vi "Timer_ISR.vi"(11 "TIMX_Interrupt":T1) -> ()   [LabVIEW 2011]
uses:
  D:/National Instruments/LabVIEW 2011/Targets/Keil/Embedded/RealView/Generic/My_ARM_Starter_Board_F4/STM32_DriverVI_Interface/Timer/Timer_ISR_F4.ctl
  <vilib>/eio/EIO_TerminalDirection.ctl
  <vilib>/STM32_DriverVI_Interface_F4/Timer/TIM5_Flag_F4.ctl
  <vilib>/STM32_DriverVI_Interface_F4/Timer/TIM5_Capture_Channel_F4.ctl
  <vilib>/STM32_DriverVI_Interface_F4/Timer/Edge Mode_F4.ctl
  <vilib>/STM32_DriverVI_Interface_F4/Timer/TIM5_Get_Channel_F4.ctl
  <vilib>/STM32_DriverVI_Interface_F4/GPIO_EIO/GPO_EIO_Inner_F4.vi
  <vilib>/STM32_DriverVI_Interface_F4/Timer/Clear_TIM5_Flag_F4.vi
  <vilib>/STM32_DriverVI_Interface_F4/Timer/TIM5 Channel Edge Set_F4.vi
  <vilib>/STM32_DriverVI_Interface_F4/Timer/TIM5_Set_Counter_F4.vi
  <vilib>/STM32_DriverVI_Interface_F4/Timer/TIM5 Get Channel_Value_F4.vi
  <vilib>/eio/EIONode/EIONode.xnode
panel:
  # "这是一个标准的中断模板 VI，用户可以直接使用,\n在相应的Case语句里面实现相应的中断服务程序即可！\n\n双击打开这个VI之后，另存为副本，名称不变，将其保存\n并添加到项目浏览器中，然后在程序生成规范中进行属性\n设置！"
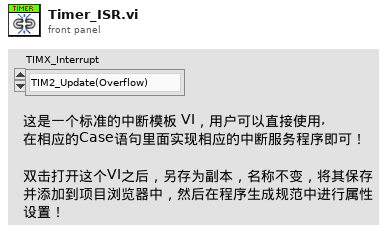
[diagram p1: front panel]
types:
  T1 = typedef "Timer_ISR_F4.ctl" = enum8{"TIM2_Update(Overflow)", "TIM2_Channel_1", "TIM2_Channel_2", "TIM2_Channel_3", "TIM2_Channel_4", "TIM3_Update(Overflow)", "TIM3_Channel_1", "TIM3_Channel_2", "TIM3_Channel_3", "TIM3_Channel_4", "TIM4_Update(Overflow)", "TIM4_Channel_1", "TIM4_Channel_2", "TIM4_Channel_3", "TIM4_Channel_4", "TIM5_Update(Overflow)", "TIM5_Channel_1", "TIM5_Channel_2", "TIM5_Channel_3", "TIM5_Channel_4", "TIM6_Update(Overflow)", "TIM7_Update(Overflow)", "----------------------------", "WWDG_ISR", "RTC_Alarm_ClockA_ISR", "RTC_Alarm_ClockB_ISR", "RTC_WKUP_ISR", "TIM1_Update(Overflow)", "TIM1_Channel_1", "TIM1_Channel_2", "TIM1_Channel_3", "TIM1_Channel_4", "TIM8_Update(Overflow)", "TIM8_Channel_1", "TIM8_Channel_2", "TIM8_Channel_3", "TIM8_Channel_4", "TIM9_Update(Overflow)", "TIM9_Channel_1", "TIM9_Channel_2", "TIM10_Update(Overflow)", "TIM10_Channel_1", "TIM11_Update(Overflow)", "TIM11_Channel_1", "TIM12_Update(Overflow)", "TIM12_Channel_1", "TIM12_Channel_2", "TIM13_Update(Overflow)", "TIM13_Channel_1", "TIM14_Update(Overflow)", "TIM14_Channel_1"}
  T2 = enum8{"P0", "P1", "P2", "P3", "P4", "P5", "P6", "P7", "P8", "P9", "P10", "P11", "P12", "P13", "P14", "P15"}
  T3 = typedef "TIM5_Flag_F4.ctl" = enum8{"TIM5_Update(Overflow)", "TIM5_Channel_1", "TIM5_Channel_2", "TIM5_Channel_3", "TIM5_Channel_4", "TIM5_Reserved……", "TIM5_Trigger(Pulse)"}
  T4 = typedef "TIM5_Capture_Channel_F4.ctl" = enum8{"TIM5_Channel_1", "TIM5_Channel_2", "TIM5_Channel_3", "TIM5_Channel_4"}
  T5 = typedef "Edge Mode_F4.ctl" = enum8{"Rising edge", "Falling edge"}
  T6 = typedef "TIM5_Get_Channel_F4.ctl" = enum8{"TIM5_Channel_1", "TIM5_Channel_2", "TIM5_Channel_3", "TIM5_Channel_4"}
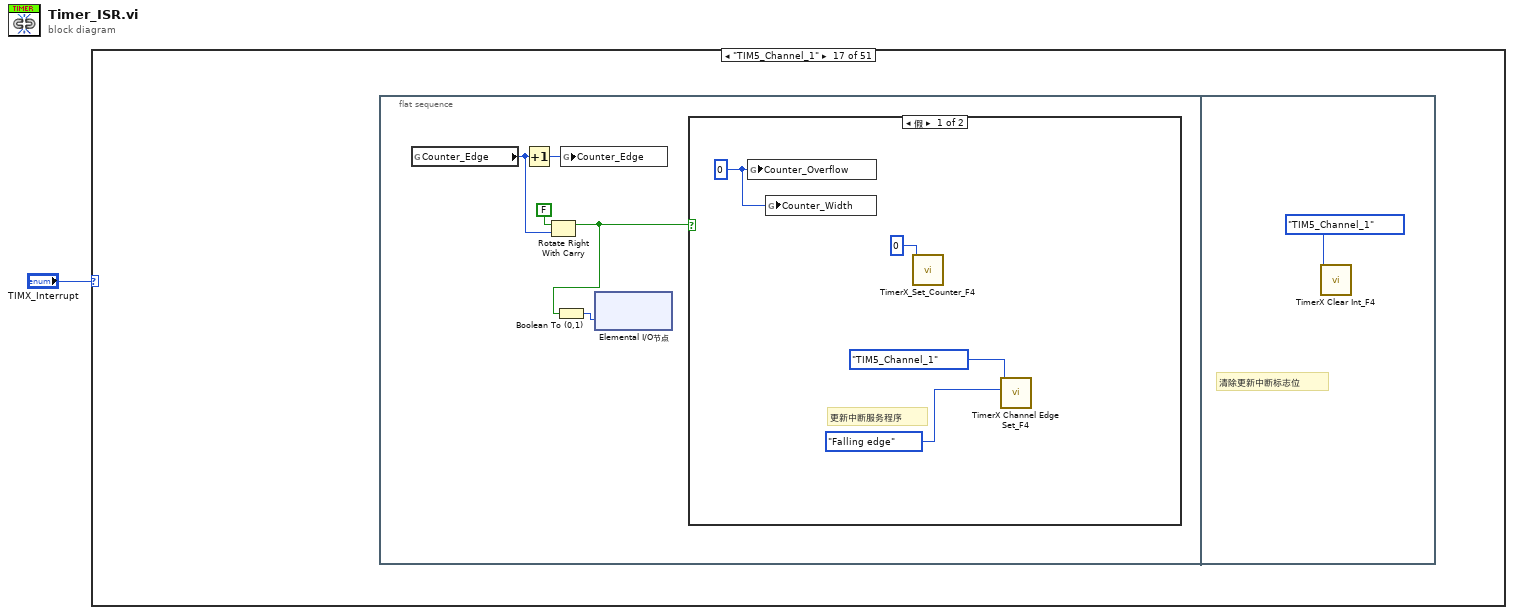
[diagram p0: block diagram]
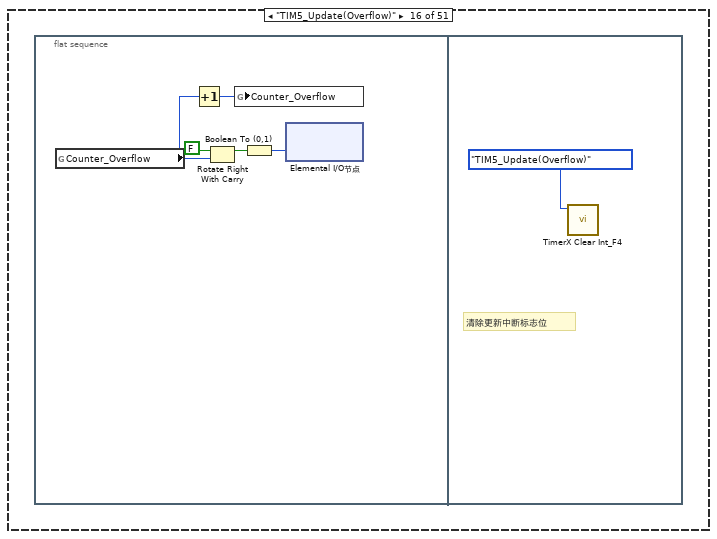
[diagram p17: hidden frame]
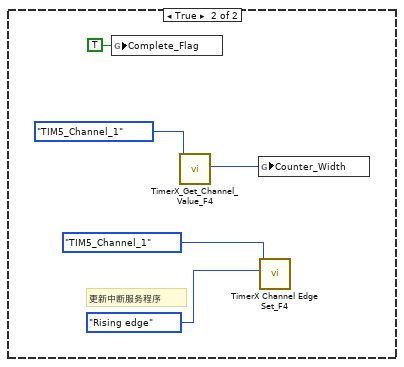
[diagram p18: hidden frame]
diagram:
  n1 = case shown="\"TIM5_Channel_1\"" "TIMX_Interrupt" {
    frame "TIM2_Update(Overflow)", Default {
    }
    frame "TIM2_Channel_1" {
    }
    frame "TIM2_Channel_2" {
      # "一个中断号只对应一个引脚中断时，直接处理"
    }
    frame "TIM2_Channel_3" {
    }
    frame "TIM2_Channel_4" {
    }
    frame "TIM3_Update(Overflow)" {
    }
    frame "TIM3_Channel_1" {
    }
    frame "TIM3_Channel_2" {
    }
    frame "TIM3_Channel_3" {
    }
    frame "TIM3_Channel_4" {
    }
    frame "TIM4_Update(Overflow)" {
    }
    frame "TIM4_Channel_1" {
    }
    frame "TIM4_Channel_2" {
    }
    frame "TIM4_Channel_3" {
    }
    frame "TIM4_Channel_4" {
    }
    frame "TIM5_Update(Overflow)" {
      n2 = flat-sequence {
        frame #0 {
          n3 = global read "全局变量.vi" "Counter_Overflow"() -> (w5:i32)
          n4 = Increment(x=w5) -> (x+1=w6:i32)
          n5 = Rotate Right With Carry(2:w5, 3:FALSE ("进位")) -> (1:w2:bool)  [unwired: 1 out]
          n6 = global write "全局变量.vi" "Counter_Overflow"(w6) -> ()
          n7 = Boolean To (0,1)(Boolean=w2) -> (0, 1=w3:i16)
          n8 = xnode "Elemental I/O节点"("LED_2"=w3) -> ()  [unwired: 1 in, 1 out]
        }
        frame #1 {
          # "清除更新中断标志位"
          n9 = call-poly <vilib>:"TimerX Clear Int_F4.vi"("TIM5_Flag"=TIM5_Flag_F4."TIM5_Update(Overflow)") -> ()  [unwired: 10 in, 1 out]
        }
      }
    }
    frame "TIM5_Channel_1" {
      n10 = flat-sequence {
        frame #0 {
          n11 = global read "全局变量.vi" "Counter_Edge"() -> (w15:i32)
          n12 = Increment(x=w15) -> (x+1=w16:i32)
          n13 = Rotate Right With Carry(2:w15, 3:FALSE ("进位")) -> (1:w12:bool)  [unwired: 1 out]
          n14 = Boolean To (0,1)(Boolean=w12) -> (0, 1=w13:i16)
          n15 = global write "全局变量.vi" "Counter_Edge"(w16) -> ()
          n16 = xnode "Elemental I/O节点"("LED_1"=w13) -> ()  [unwired: 1 in, 1 out]
          n17 = case shown="假" w12 {
            frame False {
              w20 = 0 ("Counter_Overflow")
              # "更新中断服务程序"
              n18 = global write "全局变量.vi" "Counter_Overflow"(w20) -> ()
              n19 = global write "全局变量.vi" "Counter_Width"(w20) -> ()
              n20 = call-poly <vilib>:"TimerX_Set_Counter_F4.vi"("Counter_Value"=u16 0) -> ()  [unwired: 10 in, 1 out]
              n21 = call-poly <vilib>:"TimerX Channel Edge Set_F4.vi"("Edge Mode"=Edge_Mode_F4."Falling edge", "TIM5_Capture_Channel"=TIM5_Capture_Channel_F4."TIM5_Channel_1") -> ()  [unwired: 9 in, 1 out]
            }
            frame True {
              # "更新中断服务程序"
              n22 = global write "全局变量.vi" "Complete_Flag"(TRUE ("Complete_Flag")) -> ()
              n23 = call-poly <vilib>:"TimerX_Get_Channel_Value_F4.vi"("TIM5_Channel"=TIM5_Get_Channel_F4."TIM5_Channel_1") -> ("Channel_Value"=w23:u16)  [unwired: 9 in, 1 out]
              n24 = global write "全局变量.vi" "Counter_Width"(w23) -> ()
              n25 = call-poly <vilib>:"TimerX Channel Edge Set_F4.vi"("Edge Mode"=Edge_Mode_F4."Rising edge", "TIM5_Capture_Channel"=TIM5_Capture_Channel_F4."TIM5_Channel_1") -> ()  [unwired: 9 in, 1 out]
            }
          }
        }
        frame #1 {
          # "清除更新中断标志位"
          n26 = call-poly <vilib>:"TimerX Clear Int_F4.vi"("TIM5_Flag"=TIM5_Flag_F4."TIM5_Channel_1") -> ()  [unwired: 10 in, 1 out]
        }
      }
    }
    frame "TIM5_Channel_2" {
    }
    frame "TIM5_Channel_3" {
    }
    frame "TIM5_Channel_4" {
    }
    frame "TIM6_Update(Overflow)" {
    }
    frame "TIM7_Update(Overflow)" {
    }
    frame "----------------------------" {
    }
    frame "WWDG_ISR" {
    }
    frame "RTC_Alarm_ClockA_ISR" {
    }
    frame "RTC_Alarm_ClockB_ISR" {
    }
    frame "RTC_WKUP_ISR" {
    }
    frame "TIM1_Update(Overflow)" {
    }
    frame "TIM1_Channel_1" {
    }
    frame "TIM1_Channel_2" {
    }
    frame "TIM1_Channel_3" {
    }
    frame "TIM1_Channel_4" {
    }
    frame "TIM8_Update(Overflow)" {
    }
    frame "TIM8_Channel_1" {
    }
    frame "TIM8_Channel_2" {
    }
    frame "TIM8_Channel_3" {
    }
    frame "TIM8_Channel_4" {
    }
    frame "TIM9_Update(Overflow)" {
    }
    frame "TIM9_Channel_1" {
    }
    frame "TIM9_Channel_2" {
    }
    frame "TIM10_Update(Overflow)" {
    }
    frame "TIM10_Channel_1" {
    }
    frame "TIM11_Update(Overflow)" {
    }
    frame "TIM11_Channel_1" {
    }
    frame "TIM12_Update(Overflow)" {
    }
    frame "TIM12_Channel_1" {
    }
    frame "TIM12_Channel_2" {
    }
    frame "TIM13_Update(Overflow)" {
    }
    frame "TIM13_Channel_1" {
    }
    frame "TIM14_Update(Overflow)" {
    }
    frame "TIM14_Channel_1" {
    }
  }
